vi "Get Waypoint type.vi"(8 "Error In":errorcluster) -> (0 "Error Out":errorcluster, 3 "Waypoint Type Out":T1)   [LabVIEW 2014]
uses:
  Missions/Controls/Waypoint Type.ctl
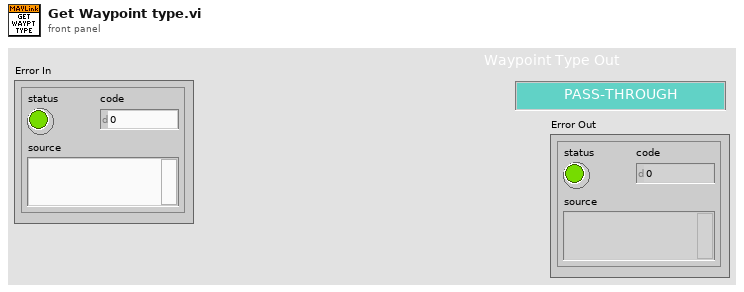
[diagram p1: front panel]
types:
  T1 = typedef "Waypoint Type.ctl" = enum16{"PASS-THROUGH", "INSPECT", "CIRCUMNAVIGATE"}
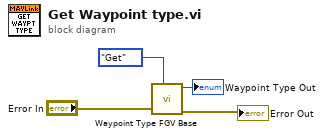
[diagram p0: block diagram]
diagram:
  n1 = call "Waypoint Type FGV Base.vi"("Method"=enum16{"Get", "Set"}."Get", "Error In"="Error In") -> ("Error Out"=→"Error Out":errorcluster, "Waypoint Type Out"=→"Waypoint Type Out":T1)  [unwired: 8 in]
